vi "RootsPumpLCW_Global.vi"() -> ()   [LabVIEW 2019]
panel:
  out "RPLCW_WFS1":dbl
  out "RPLCW_M4":dbl
  out "RPLCW_M3":dbl
  out "RPLCW_M2":dbl
  out "RPLCW_ST":u32(colorbox)
  out "RPLCW_M1":dbl
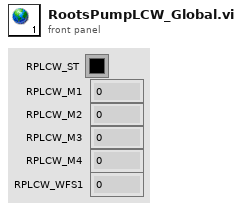
[diagram p1: front panel]
diagram:
